vi "PAQ_memory_Get_reference.vi"(8 "error in (no error)":errorcluster, 10 "PAQ_Layer":i32, 11 "FAMM in":refnum<class "FAMM.lvclass">) -> (0 "error out":errorcluster, 2 "PAQ_memory":refnum<data-value>, 3 "FAMM out":refnum<class "FAMM.lvclass">)   [LabVIEW 2020, in "FAMM.lvclass"]
doc: "Get the Reference of one PAQ memory layer"
uses:
  FAMM.lvclass
  PAQ-memory.lvclass
  FAMM.lvclass/FAMM.ctl
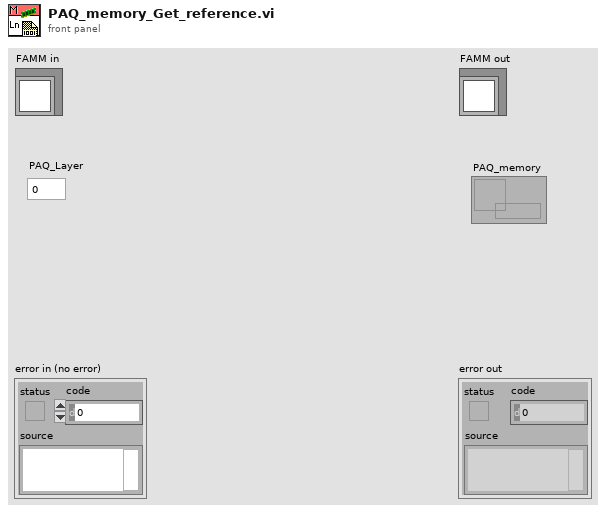
[diagram p1: front panel]
types:
  T1 = typedef "FAMM.lvclass/FAMM-attributes.ctl" = cluster{"FAMM_PAQ_Layers":i32, "FAMM_PAQ_resolution":dbl, "PAQ_TAGs":string[], "WAQ_TAGs":string[], "EAQ_TAGs":string[], "All_TAGs":string[], "PAQtagProps":T2[], "WAQtagProps":T2[], "EAQtagProps":T2[], "DBAL_class":refnum<data-value>, "PAQ_memory":refnum<data-value>[], "PAQupdates":timestamp[], "FAMM_Size":cluster{"other":i32, "1day":i32, "1week":i32}, "DatabaseFileExtention":string, "DatabaseSaveRate":dbl, "Database_path":path}
  T2 = typedef "typedef_com_TagProp.ctl" = cluster{"Description":string, "EngUnits":string, "RangeH":dbl, "RangeL":dbl, "Resolution":i32, "Obsolete":bool, "ChangeDate":timestamp, "ChangeSource":string, "ChangeReason":string, "TagFunc":u32}
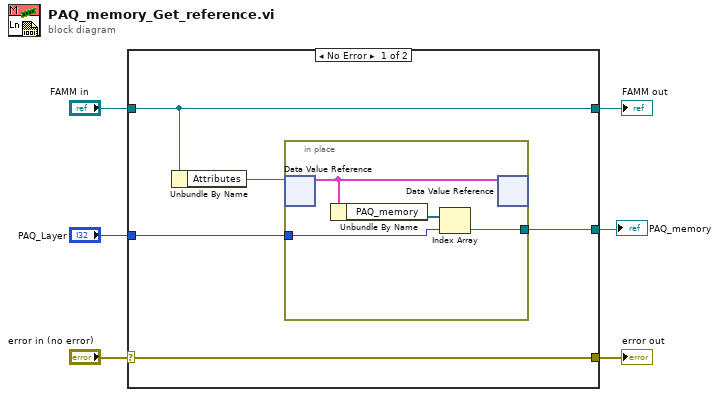
[diagram p0: block diagram]
diagram:
  n1 = case shown="No Error" "error in (no error)" {
    selector: "error in (no error)" -> [w11 w17]
    tunnel: [w11 w17] -> w5
    tunnel: [w10 w16] -> w3
    tunnel: "FAMM in" -> [w10 w16]
    tunnel: "PAQ_Layer" -> [w8 _]
    tunnel: [w7 _] -> w1
    frame No Error {
      n2 = Unbundle By Name(w10) -> ("Attributes"=w9:refnum<data-value>)
      n3 = in-place {
        in-place-border: w8 -> [w13]
        in-place-border: [w12] -> w7
        n4 = in-place-dvr #1(w9) -> (w15:T1)  [unwired: 1 out]
        n5 = Unbundle By Name(w15) -> ("PAQ_memory"=w14:refnum<data-value>[])
        n6 = Index Array(array=w14, index=w13) -> (element=w12:refnum<data-value>)
        n7 = in-place-dvr #1(w15) -> ()  [unwired: 2 out]
      }
    }
    frame Error {
    }
  }
  "error out" <- w5
  "FAMM out" <- w3
  "PAQ_memory" <- w1
